vi "Mouse PopUp Control.vi"(7 "type":T1, 8 "error in":errorcluster caption="에러 입력(에러 없음)", 9 "아이템 태그":string, 10 "Tbl 참조 번호":refnum<vi>, 11 "메뉴 참조":refnum<k9>) -> (0 "error out":errorcluster caption="에러 출력")   [LabVIEW 2020]
uses:
  Controls/Cmd_Mouse Popup.ctl
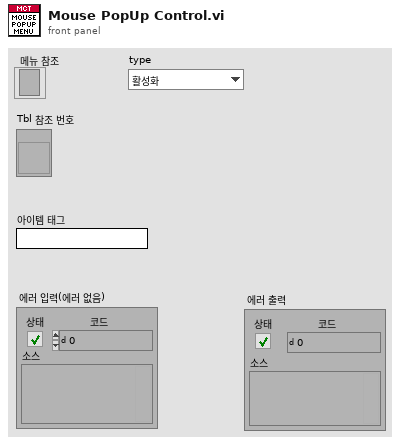
[diagram p1: front panel]
types:
  T1 = typedef "Cmd_Mouse Popup.ctl" = enum16{"활성화", "메뉴선택"}
  T2 = typedef "LVRowAndColumnTypeDef.ctl" = cluster{"Row":i32, "Column":i32}
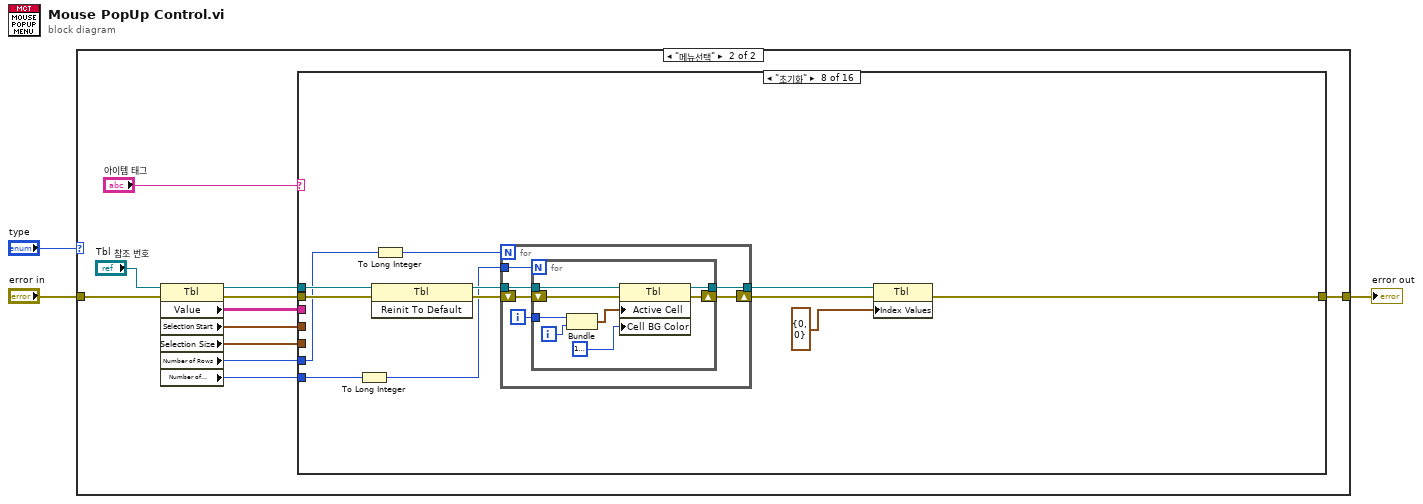
[diagram p0: block diagram]
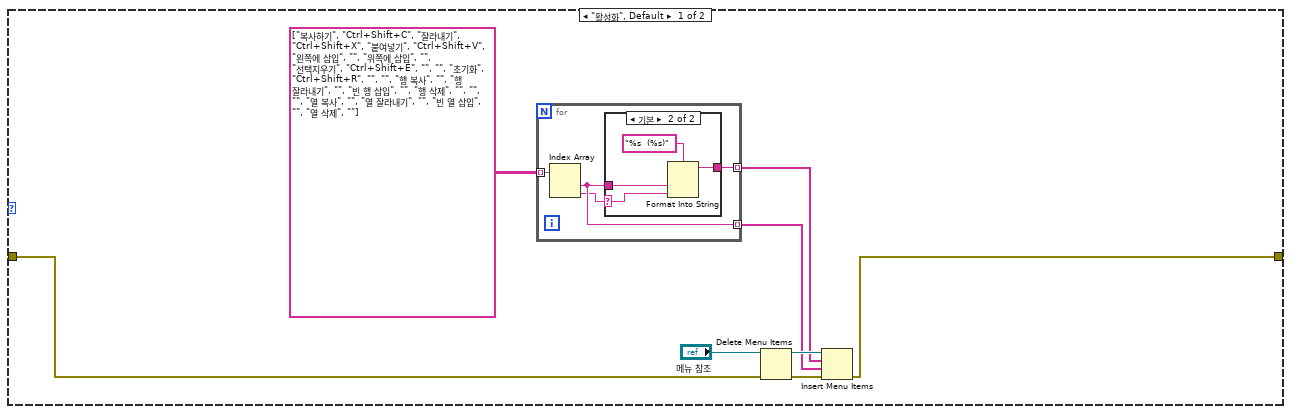
[diagram p2: hidden frame]
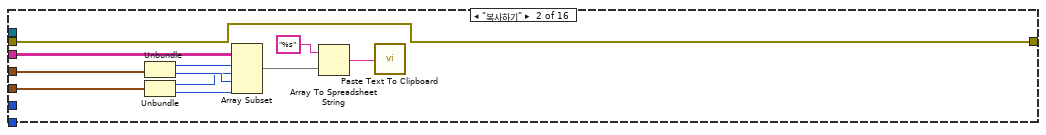
[diagram p5: hidden frame]
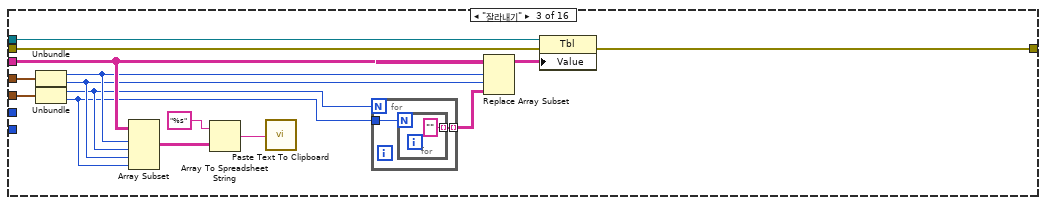
[diagram p6: hidden frame]
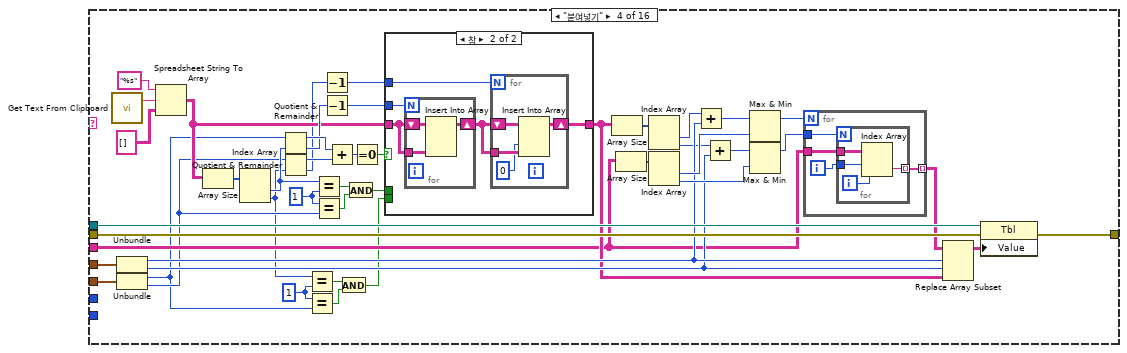
[diagram p7: hidden frame]
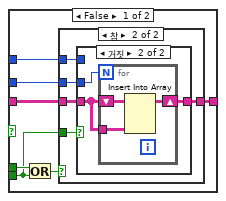
[diagram p8: hidden frame]
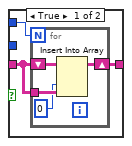
[diagram p10: hidden frame]
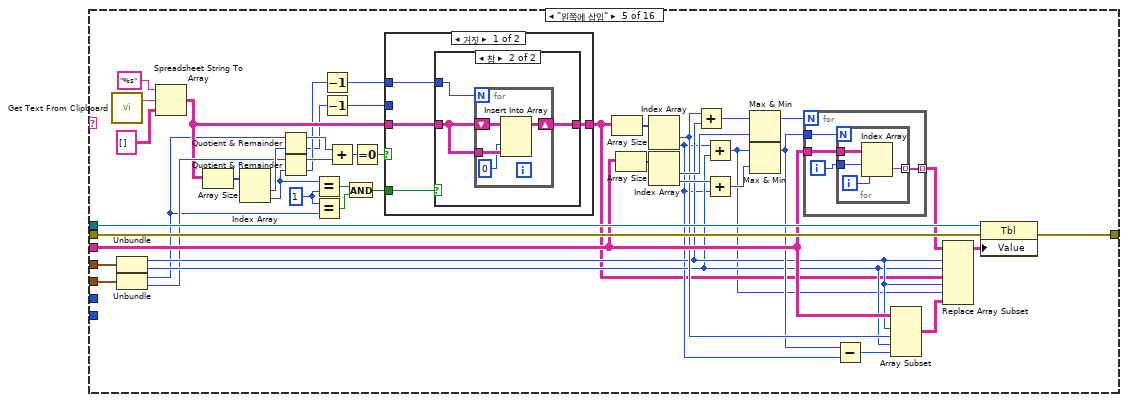
[diagram p11: hidden frame]
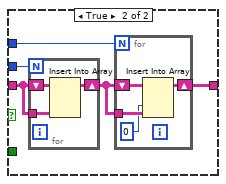
[diagram p13: hidden frame]
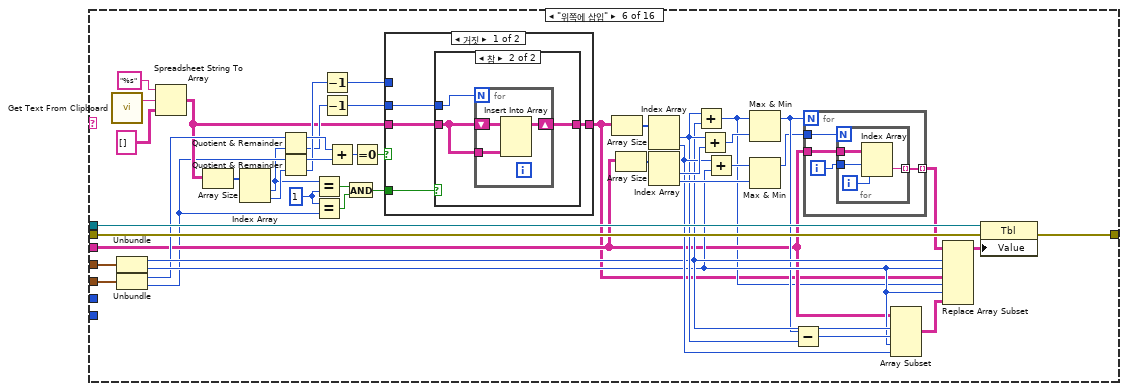
[diagram p14: hidden frame]
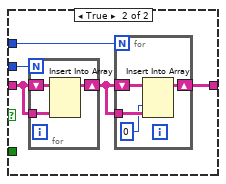
[diagram p16: hidden frame]
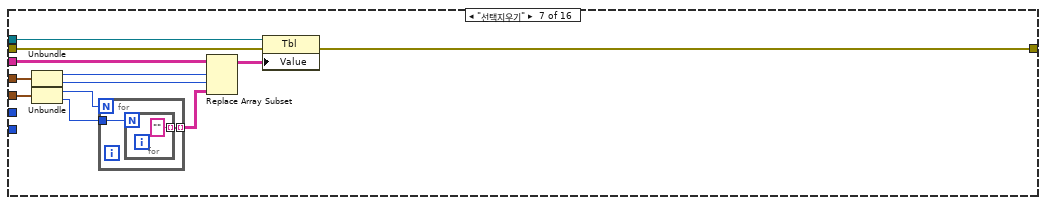
[diagram p17: hidden frame]
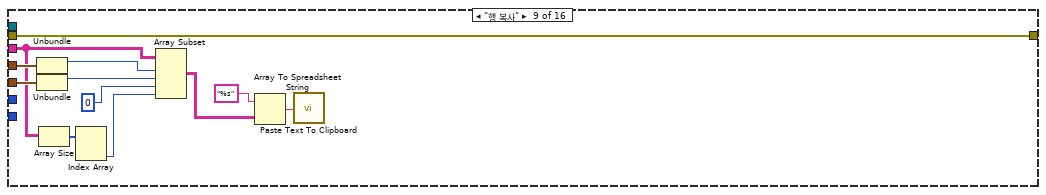
[diagram p18: hidden frame]
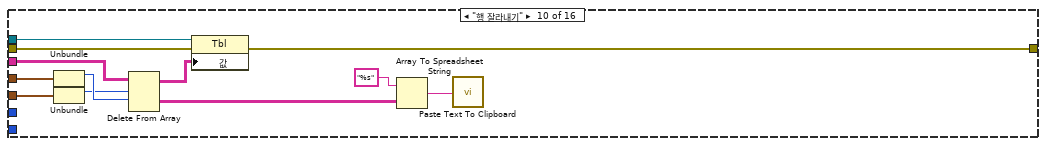
[diagram p19: hidden frame]
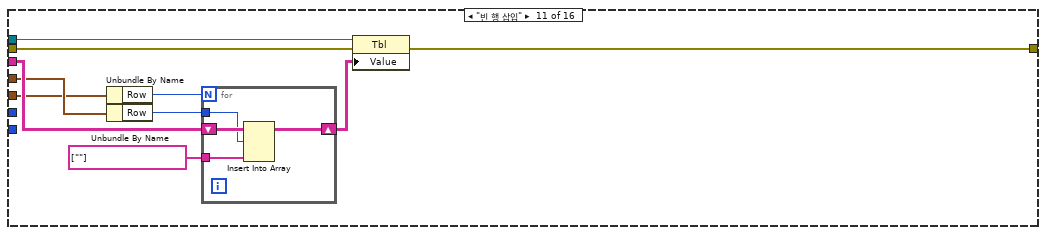
[diagram p20: hidden frame]
diagram:
  n1 = case shown="\"메뉴선택\"" "type" {
    tunnel: "error in" -> [w8 w28]
    tunnel: [w7 w30] -> w2
    frame "활성화", Default {
      n2 = for {
        tunnel: [w15] -> w6 mode=indexing
        tunnel: string[][] [["복사하기", "Ctrl+Shift+C"], ["잘라내기", "Ctrl+Shift+X"], ["붙여넣기", "Ctrl+Shift+V"], ["왼쪽에 삽입", ""], ["위쪽에 삽입", ""], ["선택지우기", "Ctrl+Shift+E"], ["", ""], ["초기화", "Ctrl+Shift+R"], ["", ""], ["행 복사", ""], ["행 잘라내기", ""], ["빈 행 삽입", ""], ["행 삭제", ""], ["", ""], ["열 복사", ""], ["열 잘라내기", ""], ["빈 열 삽입", ""], ["열 삭제", ""]] ("배열") -> [w14] mode=indexing
        tunnel: [w13] -> w4 mode=indexing
        n3 = Index Array(array=w14) -> (element #1=w13:string, element #2=w12:string)  [unwired: 2 in]
        n4 = case shown="기본" w12 {
          selector: w12 -> [_ w17]
          tunnel: [w16 w19] -> w15
          tunnel: w13 -> [w16 w18]
          frame "" {
          }
          frame Default {
            n5 = Format Into String(format string="%s  (%s)" ("포맷 문자열"), w18, w17) -> (resulting string=w19:string)  [unwired: 2 in, 1 out]
          }
        }
      }
      n6 = Delete Menu Items(6:w8, 9:"메뉴 참조") -> (0:w11:errorcluster, 3:w10:refnum<k9>)  [unwired: 2 in]
      n7 = Insert Menu Items(6:w11, 7:w4, 8:w6, 9:w10) -> (0:w7:errorcluster)  [unwired: 2 in, 2 out]
    }
    frame "메뉴선택" {
      n8 = property class="Tbl"(reference="Tbl 참조 번호", error in=w28) -> (reference out=w25:refnum<vi>, error out=w21:errorcluster, "Value"=w24:string[][], "Selection Start"=w27:T2, "Selection Size"=w26:T2, "Number of Rows"=w23:u32, "Number of Columns"=w22:u32)
      n9 = case shown="\"초기화\"" "아이템 태그" {
        tunnel: w25 -> [_ _ w56 w103 w194 w271 w307 w333 _ w361 w372 w386 _ w413 w431 w444]
        tunnel: w21 -> [w32 w43 w57 w102 w193 w270 w308 w332 w349 w362 w373 w387 w399 w414 w430 w443]
        tunnel: [w32 w43 w58 w104 w195 w272 w312 w323 w349 w368 w381 w394 w399 w419 w429 w442] -> w30
        tunnel: w24 -> [_ w35 w50 w75 w182 w245 w309 _ w350 w363 w376 w390 w400 w415 w424 w438]
        tunnel: w27 -> [_ w33 w49 w99 w190 w267 w310 _ w351 w364 w375 w389 w403 w416 w423 w437]
        tunnel: w26 -> [_ w34 w48 w91 w168 w248 w311 _ w352 w365 w374 w388 w402 w412 w422 w436]
        tunnel: w23 -> [_ _ _ _ _ _ _ w329 _ _ _ _ _ _ _ _]
        tunnel: w22 -> [_ _ _ _ _ _ _ w328 _ _ _ _ _ _ _ _]
        frame Default {
        }
        frame "복사하기" {
          n10 = Unbundle(w33) -> ("Row"=w42:i32, "Column"=w41:i32)
          n11 = Unbundle(w34) -> ("Row"=w36:i32, "Column"=w40:i32)
          n12 = Array Subset(array=w35, index (row)=w42, length (row)=w36, index (col)=w41, length (col)=w40) -> (w39:string[][])
          n13 = Array To Spreadsheet String(array=w39, 3:"%s" ("format string")) -> (spreadsheet string=w37:string)  [unwired: 1 in]
          n14 = call "Paste Text To Clipboard.vi"("Text to copy to clipboard"=w37) -> ()  [unwired: 1 out]
        }
        frame "잘라내기" {
          n15 = Unbundle(w49) -> ("Row"=w47:i32, "Column"=w46:i32)
          n16 = Unbundle(w48) -> ("Row"=w45:i32, "Column"=w44:i32)
          n17 = Array Subset(array=w50, index (row)=w47, length (row)=w45, index (col)=w46, length (col)=w44) -> (w53:string[][])
          n18 = Array To Spreadsheet String(array=w53, 3:"%s" ("format string")) -> (spreadsheet string=w51:string)  [unwired: 1 in]
          n19 = call "Paste Text To Clipboard.vi"("Text to copy to clipboard"=w51) -> ()  [unwired: 1 out]
          n20 = for {
            N: w45 -> [_]
            tunnel: w44 -> [w60]
            tunnel: [w59] -> w54 mode=indexing
            n21 = for {
              N: w60 -> [_]
              tunnel: ["" ("새 원소/부분배열")] -> w59 mode=indexing
            }
          }
          n22 = Replace Array Subset(array=w50, new element=w54, index (row)=w47, index (col)=w46) -> (w55:string[][])
          n23 = property class="Tbl"(reference=w56, error in=w57, "Value"=w55) -> (error out=w58:errorcluster)  [unwired: 1 out]
        }
        frame "붙여넣기" {
          w65 = 1 ("y")
          w73 = 1 ("y")
          n24 = call "Get Text From Clipboard.vi"() -> ("Text From Clipboard"=w106:string)  [unwired: 1 out]
          n25 = Unbundle(w99) -> ("Row"=w93:i32, "Column"=w92:i32)
          n26 = Unbundle(w91) -> ("Row"=w63:i32, "Column"=w69:i32)
          n27 = Spreadsheet String To Array(format string="%s", spreadsheet string=w106, array type (2D Dbl)=string[][] []) -> (array=w86:string[][])  [unwired: 1 in]
          n28 = Array Size(array=w86) -> (size(s)=w101:i32[])
          n29 = Index Array(array=w101) -> (element #1=w70:i32, element #2=w64:i32)  [unwired: 2 in]
          n30 = Quotient & Remainder(x=w63, y=w70) -> (x-y*floor(x/y)=w90:i32, floor(x/y)=w87:i32)
          n31 = Quotient & Remainder(x=w69, y=w64) -> (x-y*floor(x/y)=w89:i32, floor(x/y)=w79:i32)
          n32 = Equal?(x=w64, y=w65) -> (x = y?=w66:bool)
          n33 = Equal?(x=w65, y=w63) -> (x = y?=w67:bool)
          n34 = Equal?(x=w70, y=w73) -> (x = y?=w72:bool)
          n35 = Equal?(x=w73, y=w69) -> (x = y?=w71:bool)
          n36 = Decrement(x=w79) -> (x-1=w78:i32)
          n37 = Decrement(x=w87) -> (x-1=w80:i32)
          n38 = Add(x=w90, y=w89) -> (x+y=w88:i32)
          n39 = And(x=w66, y=w67) -> (x .and. y?=w62:bool)
          n40 = And(x=w72, y=w71) -> (x .and. y?=w68:bool)
          n41 = Equal To 0?(x=w88) -> (x = 0?=w85:bool)
          n42 = case shown="참" w85 {
            tunnel: w80 -> [w120 w146]
            tunnel: w86 -> [w122 w145]
            tunnel: [w119 w144] -> w83
            tunnel: w78 -> [w121 w142]
            tunnel: w68 -> [w118 _]
            tunnel: w62 -> [w117 _]
            frame False {
              n43 = Or(x=w118, y=w117) -> (x .or. y?=w116:bool)
              n44 = case shown="참" w116 {
                tunnel: w122 -> [w123 w128]
                tunnel: w117 -> [_ w127]
                tunnel: w121 -> [_ w126]
                tunnel: w120 -> [_ w125]
                tunnel: [w123 w124] -> w119
                frame False {
                }
                frame True {
                  n45 = case shown="거짓" w127 {
                    tunnel: w128 -> [w131 w138]
                    tunnel: w126 -> [w130 _]
                    tunnel: w125 -> [_ w136]
                    tunnel: [w129 w137] -> w124
                    frame True {
                      n46 = for {
                        N: w130 -> [_]
                        shift-right: [w134] -> w129
                        shift-left: w131 -> [w135]
                        tunnel: w131 -> [w133]
                        n47 = Insert Into Array(array=w135, index (col)=0 ("비활성화된 인덱스 (열)"), new element=w133) -> (w134:string[][])  [unwired: 1 in]
                      }
                    }
                    frame False {
                      n48 = for {
                        N: w136 -> [_]
                        shift-right: [w140] -> w137
                        shift-left: w138 -> [w141]
                        tunnel: w138 -> [w139]
                        n49 = Insert Into Array(array=w141, new element=w139) -> (w140:string[][])  [unwired: 2 in]
                      }
                    }
                  }
                }
              }
            }
            frame True {
              n50 = for {
                N: w146 -> [_]
                shift-right: [w151] -> w143
                shift-left: w145 -> [w153]
                tunnel: w145 -> [w152]
                n51 = Insert Into Array(array=w153, new element=w152) -> (w151:string[][])  [unwired: 2 in]
              }
              n52 = for {
                N: w142 -> [_]
                shift-right: [w148] -> w144
                shift-left: w143 -> [w150]
                tunnel: w143 -> [w149]
                n53 = Insert Into Array(array=w150, index (col)=0 ("비활성화된 인덱스 (열)"), new element=w149) -> (w148:string[][])  [unwired: 1 in]
              }
            }
          }
          n54 = Array Size(array=w83) -> (size(s)=w84:i32[])
          n55 = Array Size(array=w75) -> (size(s)=w100:i32[])
          n56 = Index Array(array=w84) -> (element #1=w82:i32, element #2=w81:i32)  [unwired: 2 in]
          n57 = Index Array(array=w100) -> (element #1=w95:i32, element #2=w94:i32)  [unwired: 2 in]
          n58 = Add(x=w82, y=w93) -> (x+y=w97:i32)
          n59 = Add(x=w81, y=w92) -> (x+y=w96:i32)
          n60 = Max & Min(x=w97, y=w95) -> (max(x,y)=w77:i32)  [unwired: 1 out]
          n61 = Max & Min(x=w96, y=w94) -> (max(x,y)=w76:i32)  [unwired: 1 out]
          n62 = for {
            N: w77 -> [_]
            tunnel: [w111] -> w74 mode=indexing
            tunnel: w76 -> [w109]
            tunnel: w75 -> [w108]
            i -> [w110]
            n63 = for {
              N: w109 -> [_]
              tunnel: [w113] -> w111 mode=indexing
              tunnel: w110 -> [w115]
              tunnel: w108 -> [w112]
              i -> [w114]
              n64 = Index Array(array=w112, index (row)=w115, index (col)=w114) -> (element=w113:string)
            }
          }
          n65 = Replace Array Subset(array=w74, new element=w83, index (row)=w93, index (col)=w92) -> (w98:string[][])
          n66 = property class="Tbl"(reference=w103, error in=w102, "Value"=w98) -> (error out=w104:errorcluster)  [unwired: 1 out]
        }
        frame "왼쪽에 삽입" {
          w157 = 1 ("y")
          n67 = call "Get Text From Clipboard.vi"() -> ("Text From Clipboard"=w197:string)  [unwired: 1 out]
          n68 = Unbundle(w190) -> ("Row"=w177:i32, "Column"=w176:i32)
          n69 = Unbundle(w168) -> ("Row"=w158:i32, "Column"=w172:i32)
          n70 = Spreadsheet String To Array(format string="%s", spreadsheet string=w197, array type (2D Dbl)=string[][] []) -> (array=w166:string[][])  [unwired: 1 in]
          n71 = Array Size(array=w166) -> (size(s)=w174:i32[])
          n72 = Index Array(array=w174) -> (element #1=w173:i32, element #2=w159:i32)  [unwired: 2 in]
          n73 = Quotient & Remainder(x=w158, y=w173) -> (x-y*floor(x/y)=w171:i32, floor(x/y)=w164:i32)
          n74 = Quotient & Remainder(x=w172, y=w159) -> (x-y*floor(x/y)=w170:i32, floor(x/y)=w165:i32)
          n75 = Equal?(x=w159, y=w157) -> (x = y?=w156:bool)
          n76 = Equal?(x=w157, y=w158) -> (x = y?=w155:bool)
          n77 = Decrement(x=w165) -> (x-1=w163:i32)
          n78 = Decrement(x=w164) -> (x-1=w162:i32)
          n79 = Add(x=w171, y=w170) -> (x+y=w169:i32)
          n80 = And(x=w156, y=w155) -> (x .and. y?=w154:bool)
          n81 = Equal To 0?(x=w169) -> (x = 0?=w167:bool)
          n82 = case shown="거짓" w167 {
            tunnel: w162 -> [_ w215]
            tunnel: w166 -> [w201 w214]
            tunnel: [w200 w213] -> w161
            tunnel: w163 -> [w199 w211]
            tunnel: w154 -> [w202 _]
            frame False {
              n83 = case shown="참" w202 {
                tunnel: w201 -> [w203 w205]
                tunnel: [w203 w206] -> w200
                tunnel: w199 -> [_ w204]
                frame False {
                }
                frame True {
                  n84 = for {
                    N: w204 -> [_]
                    shift-right: [w209] -> w206
                    shift-left: w205 -> [w210]
                    tunnel: w205 -> [w208]
                    n85 = Insert Into Array(array=w210, index (col)=0 ("비활성화된 인덱스 (열)"), new element=w208) -> (w209:string[][])  [unwired: 1 in]
                  }
                }
              }
            }
            frame True {
              n86 = for {
                N: w215 -> [_]
                shift-right: [w220] -> w212
                shift-left: w214 -> [w222]
                tunnel: w214 -> [w221]
                n87 = Insert Into Array(array=w222, new element=w221) -> (w220:string[][])  [unwired: 2 in]
              }
              n88 = for {
                N: w211 -> [_]
                shift-right: [w217] -> w213
                shift-left: w212 -> [w219]
                tunnel: w212 -> [w218]
                n89 = Insert Into Array(array=w219, index (col)=0 ("비활성화된 인덱스 (열)"), new element=w218) -> (w217:string[][])  [unwired: 1 in]
              }
            }
          }
          n90 = Array Size(array=w161) -> (size(s)=w192:i32[])
          n91 = Array Size(array=w182) -> (size(s)=w191:i32[])
          n92 = Index Array(array=w192) -> (element #1=w181:i32, element #2=w175:i32)  [unwired: 2 in]
          n93 = Index Array(array=w191) -> (element #1=w183:i32, element #2=w187:i32)  [unwired: 2 in]
          n94 = Add(x=w181, y=w177) -> (x+y=w184:i32)
          n95 = Add(x=w175, y=w176) -> (x+y=w160:i32)
          n96 = Add(x=w187, y=w175) -> (x+y=w186:i32)
          n97 = Max & Min(x=w184, y=w183) -> (max(x,y)=w185:i32)  [unwired: 1 out]
          n98 = Max & Min(x=w160, y=w186) -> (max(x,y)=w180:i32)  [unwired: 1 out]
          n99 = for {
            N: w185 -> [_]
            tunnel: [w226] -> w188 mode=indexing
            tunnel: w180 -> [w224]
            tunnel: w182 -> [w223]
            i -> [w225]
            n100 = for {
              N: w224 -> [_]
              tunnel: [w228] -> w226 mode=indexing
              tunnel: w225 -> [w230]
              tunnel: w223 -> [w227]
              i -> [w229]
              n101 = Index Array(array=w227, index (row)=w230, index (col)=w229) -> (element=w228:string)
            }
          }
          n102 = Subtract(x=w180, y=w175) -> (x-y=w179:i32)
          n103 = Array Subset(array=w182, index (row)=w177, length (row)=w181, index (col)=w176, length (col)=w179) -> (w178:string[][])
          n104 = Replace Array Subset(array=w188, new element #1=w161, index (row) #1=w177, index (col) #1=w176, new element #2=w178, index (row) #2=w177, index (col) #2=w160) -> (w189:string[][])
          n105 = property class="Tbl"(reference=w194, error in=w193, "Value"=w189) -> (error out=w195:errorcluster)  [unwired: 1 out]
        }
        frame "위쪽에 삽입" {
          w237 = 1 ("y")
          n106 = call "Get Text From Clipboard.vi"() -> ("Text From Clipboard"=w274:string)  [unwired: 1 out]
          n107 = Unbundle(w267) -> ("Row"=w257:i32, "Column"=w256:i32)
          n108 = Unbundle(w248) -> ("Row"=w254:i32, "Column"=w232:i32)
          n109 = Spreadsheet String To Array(format string="%s", spreadsheet string=w274, array type (2D Dbl)=string[][] []) -> (array=w242:string[][])  [unwired: 1 in]
          n110 = Array Size(array=w242) -> (size(s)=w255:i32[])
          n111 = Index Array(array=w255) -> (element #1=w231:i32, element #2=w234:i32)  [unwired: 2 in]
          n112 = Quotient & Remainder(x=w254, y=w231) -> (x-y*floor(x/y)=w253:i32, floor(x/y)=w249:i32)
          n113 = Quotient & Remainder(x=w232, y=w234) -> (x-y*floor(x/y)=w252:i32, floor(x/y)=w250:i32)
          n114 = Equal?(x=w231, y=w237) -> (x = y?=w236:bool)
          n115 = Equal?(x=w237, y=w232) -> (x = y?=w235:bool)
          n116 = Decrement(x=w250) -> (x-1=w239:i32)
          n117 = Decrement(x=w249) -> (x-1=w240:i32)
          n118 = Add(x=w253, y=w252) -> (x+y=w251:i32)
          n119 = And(x=w236, y=w235) -> (x .and. y?=w233:bool)
          n120 = Equal To 0?(x=w251) -> (x = 0?=w238:bool)
          n121 = case shown="거짓" w238 {
            tunnel: w240 -> [w276 w291]
            tunnel: w242 -> [w278 w290]
            tunnel: [w277 w289] -> w241
            tunnel: w239 -> [_ w287]
            tunnel: w233 -> [w279 _]
            frame False {
              n122 = case shown="참" w279 {
                tunnel: w278 -> [w280 w283]
                tunnel: [w280 w282] -> w277
                tunnel: w276 -> [_ w281]
                frame False {
                }
                frame True {
                  n123 = for {
                    N: w281 -> [_]
                    shift-right: [w285] -> w282
                    shift-left: w283 -> [w286]
                    tunnel: w283 -> [w284]
                    n124 = Insert Into Array(array=w286, new element=w284) -> (w285:string[][])  [unwired: 2 in]
                  }
                }
              }
            }
            frame True {
              n125 = for {
                N: w291 -> [_]
                shift-right: [w296] -> w288
                shift-left: w290 -> [w298]
                tunnel: w290 -> [w297]
                n126 = Insert Into Array(array=w298, new element=w297) -> (w296:string[][])  [unwired: 2 in]
              }
              n127 = for {
                N: w287 -> [_]
                shift-right: [w293] -> w289
                shift-left: w288 -> [w295]
                tunnel: w288 -> [w294]
                n128 = Insert Into Array(array=w295, index (col)=0 ("비활성화된 인덱스 (열)"), new element=w294) -> (w293:string[][])  [unwired: 1 in]
              }
            }
          }
          n129 = Array Size(array=w241) -> (size(s)=w269:i32[])
          n130 = Array Size(array=w245) -> (size(s)=w268:i32[])
          n131 = Index Array(array=w269) -> (element #1=w259:i32, element #2=w260:i32)  [unwired: 2 in]
          n132 = Index Array(array=w268) -> (element #1=w262:i32, element #2=w261:i32)  [unwired: 2 in]
          n133 = Add(x=w259, y=w257) -> (x+y=w243:i32)
          n134 = Add(x=w259, y=w262) -> (x+y=w263:i32)
          n135 = Add(x=w260, y=w256) -> (x+y=w265:i32)
          n136 = Max & Min(x=w243, y=w263) -> (max(x,y)=w247:i32)  [unwired: 1 out]
          n137 = Max & Min(x=w265, y=w261) -> (max(x,y)=w246:i32)  [unwired: 1 out]
          n138 = Subtract(x=w247, y=w259) -> (x-y=w258:i32)
          n139 = for {
            N: w247 -> [_]
            tunnel: [w302] -> w244 mode=indexing
            tunnel: w246 -> [w300]
            tunnel: w245 -> [w299]
            i -> [w301]
            n140 = for {
              N: w300 -> [_]
              tunnel: [w304] -> w302 mode=indexing
              tunnel: w301 -> [w306]
              tunnel: w299 -> [w303]
              i -> [w305]
              n141 = Index Array(array=w303, index (row)=w306, index (col)=w305) -> (element=w304:string)
            }
          }
          n142 = Array Subset(array=w245, index (row)=w257, length (row)=w258, index (col)=w256, length (col)=w260) -> (w264:string[][])
          n143 = Replace Array Subset(array=w244, new element #1=w241, index (row) #1=w257, index (col) #1=w256, new element #2=w264, index (row) #2=w243, index (col) #2=w256) -> (w266:string[][])
          n144 = property class="Tbl"(reference=w271, error in=w270, "Value"=w266) -> (error out=w272:errorcluster)  [unwired: 1 out]
        }
        frame "선택지우기" {
          n145 = Unbundle(w310) -> ("Row"=w317:i32, "Column"=w316:i32)
          n146 = Unbundle(w311) -> ("Row"=w314:i32, "Column"=w313:i32)
          n147 = for {
            N: w314 -> [_]
            tunnel: w313 -> [w320]
            tunnel: [w319] -> w315 mode=indexing
            n148 = for {
              N: w320 -> [_]
              tunnel: ["" ("새 원소/부분배열")] -> w319 mode=indexing
            }
          }
          n149 = Replace Array Subset(array=w309, new element=w315, index (row)=w317, index (col)=w316) -> (w318:string[][])
          n150 = property class="Tbl"(reference=w307, error in=w308, "Value"=w318) -> (error out=w312:errorcluster)  [unwired: 1 out]
        }
        frame "초기화" {
          n151 = To Long Integer(number=w328) -> (32bit integer=w326:i32)
          n152 = invoke class="Tbl" method="Reinit To Default"(reference=w333, error in=w332) -> (reference out=w330:refnum<vi>, error out=w331:errorcluster)  [unwired: 1 in, 1 out]
          n153 = To Long Integer(number=w329) -> (32bit integer=w327:i32)
          n154 = for {
            N: w327 -> [_]
            tunnel: w330 -> [w338]
            shift-right: [w337] -> w325
            shift-left: w331 -> [w339]
            tunnel: w326 -> [w335]
            tunnel: [w334] -> w324
            i -> [w336]
            n155 = for {
              N: w335 -> [_]
              tunnel: w338 -> [w346]
              shift-right: [w345] -> w337
              shift-left: w339 -> [w347]
              tunnel: w336 -> [w343]
              tunnel: [w340] -> w334
              i -> [w342]
              n156 = Bundle(w343, w342) -> (w344:cluster{i32, i32})  [unwired: 1 in]
              n157 = property class="Tbl"(reference=w346, error in=w347, "Active Cell"=w344, "Cell BG Color"=u32 16777226) -> (reference out=w340:refnum<vi>, error out=w345:errorcluster)
            }
          }
          n158 = property class="Tbl"(reference=w324, error in=w325, "Index Values"=cluster{i32, i32} {0, 0}) -> (error out=w323:errorcluster)  [unwired: 1 out]
        }
        frame "행 복사" {
          n159 = Unbundle(w351) -> ("Row"=w355:i32)  [unwired: 1 out]
          n160 = Unbundle(w352) -> ("Row"=w354:i32)  [unwired: 1 out]
          n161 = Array Size(array=w350) -> (size(s)=w357:i32[])
          n162 = Index Array(array=w357) -> (element #2=w356:i32)  [unwired: 2 in, 1 out]
          n163 = Array Subset(array=w350, index (row)=w355, length (row)=w354, index (col)=0 ("인덱스"), length (col)=w356) -> (w348:string[][])
          n164 = Array To Spreadsheet String(array=w348, 3:"%s" ("format string")) -> (spreadsheet string=w358:string)  [unwired: 1 in]
          n165 = call "Paste Text To Clipboard.vi"("Text to copy to clipboard"=w358) -> ()  [unwired: 1 out]
        }
        frame "행 잘라내기" {
          n166 = Unbundle(w364) -> ("Row"=w369:i32)  [unwired: 1 out]
          n167 = Unbundle(w365) -> ("Row"=w360:i32)  [unwired: 1 out]
          n168 = Delete From Array(array=w363, length=w360, index (row)=w369) -> (deleted portion=w366:string[][], array with subset deleted=w367:string[][])  [unwired: 1 in]
          n169 = property class="Tbl"(reference=w361, error in=w362, "값"=w367) -> (error out=w368:errorcluster)  [unwired: 1 out]
          n170 = Array To Spreadsheet String(array=w366, 3:"%s" ("format string")) -> (spreadsheet string=w370:string)  [unwired: 1 in]
          n171 = call "Paste Text To Clipboard.vi"("Text to copy to clipboard"=w370) -> ()  [unwired: 1 out]
        }
        frame "빈 행 삽입" {
          n172 = Unbundle By Name(w374) -> ("Row"=w377:i32)
          n173 = Unbundle By Name(w375) -> ("Row"=w380:i32)
          n174 = for {
            N: w377 -> [_]
            tunnel: w380 -> [w384]
            tunnel: string[] [""] ("새 원소/부분배열") -> [w383]
            shift-right: [w382] -> w378
            shift-left: w376 -> [w385]
            n175 = Insert Into Array(array=w385, index (row)=w384, new element=w383) -> (w382:string[][])  [unwired: 1 in]
          }
          n176 = property on="Property Node" class="Tbl"(reference=w372, error in=w373, "Value"=w378) -> (error out=w381:errorcluster)  [unwired: 1 out]
        }
        frame "행 삭제" {
          n177 = Unbundle By Name(w388) -> ("Row"=w393:i32)
          n178 = Unbundle By Name(w389) -> ("Row"=w392:i32)
          n179 = for {
            N: w393 -> [_]
            tunnel: w392 -> [w397]
            shift-right: [w395] -> w391
            shift-left: w390 -> [w396]
            n180 = Delete From Array(array=w396, index (row)=w397) -> (array with subset deleted=w395:string[][])  [unwired: 2 in, 1 out]
          }
          n181 = property on="Property Node" class="Tbl"(reference=w386, error in=w387, "Value"=w391) -> (error out=w394:errorcluster)  [unwired: 1 out]
        }
        frame "열 복사" {
          n182 = Array Size(array=w400) -> (size(s)=w407:i32[])
          n183 = Unbundle(w403) -> ("Column"=w406:i32)  [unwired: 1 out]
          n184 = Unbundle(w402) -> ("Column"=w401:i32)  [unwired: 1 out]
          n185 = Index Array(array=w407) -> (element #1=w404:i32)  [unwired: 2 in, 1 out]
          n186 = Array Subset(array=w400, index (row)=0 ("인덱스"), length (row)=w404, index (col)=w406, length (col)=w401) -> (w398:string[][])
          n187 = Array To Spreadsheet String(array=w398, 3:"%s" ("format string")) -> (spreadsheet string=w408:string)  [unwired: 1 in]
          n188 = call "Paste Text To Clipboard.vi"("Text to copy to clipboard"=w408) -> ()  [unwired: 1 out]
        }
        frame "열 잘라내기" {
          n189 = Unbundle(w416) -> ("Column"=w417:i32)  [unwired: 1 out]
          n190 = Unbundle(w412) -> ("Column"=w411:i32)  [unwired: 1 out]
          n191 = Delete From Array(array=w415, length=w411, index (col)=w417) -> (deleted portion=w410:string[][], array with subset deleted=w418:string[][])  [unwired: 1 in]
          n192 = property class="Tbl"(reference=w413, error in=w414, "값"=w418) -> (error out=w419:errorcluster)  [unwired: 1 out]
          n193 = Array To Spreadsheet String(array=w410, 3:"%s" ("format string")) -> (spreadsheet string=w420:string)  [unwired: 1 in]
          n194 = call "Paste Text To Clipboard.vi"("Text to copy to clipboard"=w420) -> ()  [unwired: 1 out]
        }
        frame "빈 열 삽입" {
          n195 = Unbundle By Name(w422) -> ("Column"=w425:i32)
          n196 = Unbundle By Name(w423) -> ("Column"=w426:i32)
          n197 = for {
            N: w425 -> [_]
            tunnel: string[] [""] ("새 원소/부분배열") -> [w434]
            tunnel: w426 -> [w432]
            shift-right: [w433] -> w427
            shift-left: w424 -> [w435]
            n198 = Insert Into Array(array=w435, index (col)=w432, new element=w434) -> (w433:string[][])  [unwired: 1 in]
          }
          n199 = property on="Property Node" class="Tbl"(reference=w431, error in=w430, "Value"=w427) -> (error out=w429:errorcluster)  [unwired: 1 out]
        }
        frame "열 삭제" {
          n200 = Unbundle By Name(w436) -> ("Column"=w441:i32)
          n201 = Unbundle By Name(w437) -> ("Column"=w440:i32)
          n202 = for {
            N: w441 -> [_]
            tunnel: w440 -> [w445]
            shift-right: [w446] -> w439
            shift-left: w438 -> [w447]
            n203 = Delete From Array(array=w447, index (col)=w445) -> (array with subset deleted=w446:string[][])  [unwired: 2 in, 1 out]
          }
          n204 = property on="Property Node" class="Tbl"(reference=w444, error in=w443, "Value"=w439) -> (error out=w442:errorcluster)  [unwired: 1 out]
        }
      }
    }
  }
  "error out" <- w2
